vi "Reset Do.vi"(8 "error in (no error)":errorcluster, 11 "Instrument in":refnum<class "DMM.NI.lvclass">) -> (0 "error out":errorcluster, 3 "Instrument out":refnum<class "DMM.NI.lvclass">)   [LabVIEW 2020, in "NI DMM Driver.lvlib" / "DMM.NI.lvclass"]
doc: "Reset the Instrument."
uses:
  DMM.NI.lvclass
  PPL/HDH.Driver.DMM.lvlibp/DMM Driver.lvclass
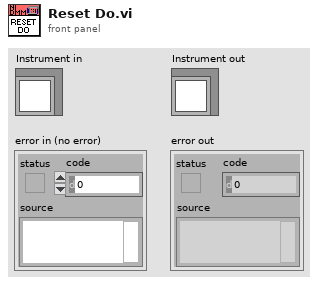
[diagram p1: front panel]
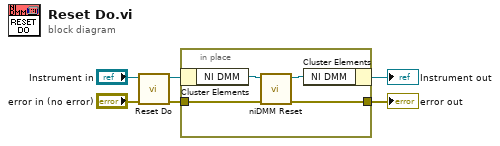
[diagram p0: block diagram]
diagram:
  n1 = call-parent "Reset Do.vi"("error in (no error)"="error in (no error)", "Instrument in"="Instrument in") -> ("error out"=w2:errorcluster, "Instrument out"=w4:refnum<class "DMM.NI.lvclass">)  [unwired: 8 in]
  n2 = in-place {
    in-place-border: w2 -> [w8]
    in-place-border: [w7] -> w1
    n3 = in-place-cluster #1(w4) -> ("NI DMM"=w10:refnum<k15>)
    n4 = call <instrlib>:"niDMM Reset.vi"("error in (no error)"=w8, "instrument handle"=w10) -> ("error out"=w7:errorcluster, "instrument handle out"=w9:refnum<k15>)  [unwired: 8 in]
    n5 = in-place-cluster #1("NI DMM"=w9) -> (→"Instrument out":refnum<class "DMM.NI.lvclass">)
  }
  "error out" <- w1
